vi "ADI_IMU_ADIS16448_AHRS_Madgwick.vi"(6 "Yaw Axis":enum16{"X", "Y", "Z"}(ring)=enum."Z", 8 "Reset?":bool, 9 "delta t":dbl, 10 "Beta":dbl, 11 "Data":dbl[](array[numeric])) -> (3 "Output":cluster{"Pitch":dbl, "Roll":dbl, "Yaw":dbl})   [LabVIEW 2019, in "ADIS16448_IMU.lvlib"]
uses:
  ADIS16448_IMU.lvlib
panel:
  out "Quaternion":dbl[](array[numeric])
  out "Pitch":dbl
  out "Roll":dbl
  out "Yaw":dbl
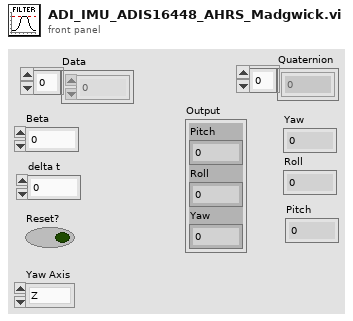
[diagram p1: front panel]
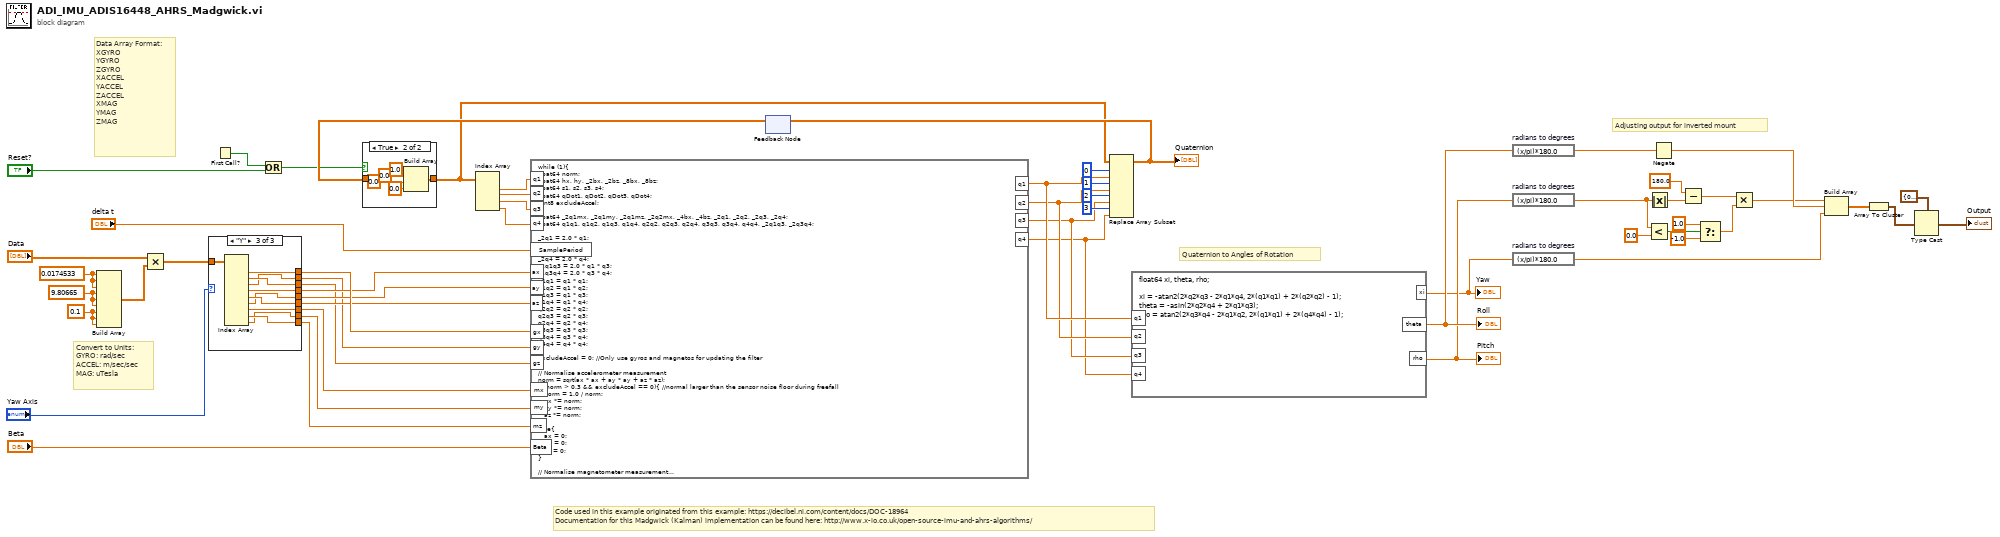
[diagram p0: block diagram]
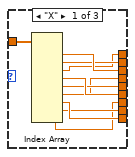
[diagram p2: hidden frame]
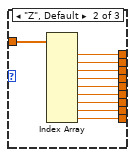
[diagram p3: hidden frame]
diagram:
  w50 = 0.1
  w51 = 9.80665
  w52 = 0.0174533
  # "Code used in this example originated from this example: https://decibel.ni.com/content/docs/DOC-18964\nDocumentation for this Madgwick (Kalman) implementation can be found here: http://www.x-io.co.uk/open-source-imu-and-ahrs-algorithms/"
  # "Quaternion to Angles of Rotation"
  # "Convert to Units:\nGYRO: rad/sec\nACCEL: m/sec/sec\nMAG: uTesla"
  # "Data Array Format:\nXGYRO\nYGYRO\nZGYRO\nXACCEL\nYACCEL\nZACCEL\nXMAG\nYMAG\nZMAG"
  # "Adjusting output for inverted mount"
  n1 = Build Array(w52, w52, w52, w51, w51, w51, w50, w50, w50) -> (w53:dbl[])
  n2 = Multiply(x="Data", y=w53) -> (x*y=w49:dbl[])
  n3 = case shown="\"Y\"" "Yaw Axis" {
    tunnel: [w63 w76 w85] -> w56
    tunnel: [w60 w75 w82] -> w55
    tunnel: w49 -> [w66 w74 w86]
    tunnel: [w57 w73 w79] -> w26
    tunnel: [w61 w72 w80] -> w25
    tunnel: [w62 w71 w81] -> w24
    tunnel: [w64 w70 w83] -> w23
    tunnel: [w65 w69 w84] -> w22
    tunnel: [w58 w68 w77] -> w21
    tunnel: [w59 w67 w78] -> w20
    frame "X" {
      n4 = Index Array(array=w66) -> (element #1=w65:dbl, element #2=w64:dbl, element #3=w63:dbl, element #4=w62:dbl, element #5=w61:dbl, element #6=w60:dbl, element #7=w59:dbl, element #8=w58:dbl, element #9=w57:dbl)  [unwired: 9 in]
    }
    frame "Z", Default {
      n5 = Index Array(array=w74) -> (element #1=w76:dbl, element #2=w70:dbl, element #3=w69:dbl, element #4=w75:dbl, element #5=w72:dbl, element #6=w71:dbl, element #7=w73:dbl, element #8=w68:dbl, element #9=w67:dbl)  [unwired: 9 in]
    }
    frame "Y" {
      n6 = Index Array(array=w86) -> (element #1=w85:dbl, element #2=w84:dbl, element #3=w83:dbl, element #4=w82:dbl, element #5=w81:dbl, element #6=w80:dbl, element #7=w79:dbl, element #8=w78:dbl, element #9=w77:dbl)  [unwired: 9 in]
    }
  }
  n7 = First Call?() -> (First Call?: T/F=w32:bool)
  n8 = Or(x=w32, y="Reset?") -> (x .or. y?=w33:bool)
  n9 = feedback #1() -> (w35:dbl[])  [unwired: 1 in]
  n10 = case shown="True" w33 {
    tunnel: w35 -> [w87 _]
    tunnel: [w87 w88] -> w34
    frame False {
    }
    frame True {
      n11 = Build Array(1.0 ("element"), 0.0 ("element"), 0.0 ("element"), 0.0 ("element")) -> (w88:dbl[])
    }
  }
  n12 = Index Array(array=w34) -> (element #1=w48:dbl, element #2=w47:dbl, element #3=w46:dbl, element #4=w45:dbl)  [unwired: 4 in]
  n13 = formula code="while (1){\nfloat64 norm;\nfloat64 hx, hy, _2bx, _2bz, _8bx, _8bz;\nfloat64 s1, s2, s3, s4;\nfloat64 qDot1, qDot2, qDot3, qDot4;\nuInt8 excludeAccel;\n\nfloat64 _2q1mx, _2q1my, _2q1mz, _2q2mx, _4bx, _4bz, _2q1, _2q2, _2q3, _2q4;\nfloat64 q1q1, q1q2, q1q3, q1q4, q2q2, q2q3, q2q4, q3q3, q3q4, q4q4, _2q1q3, _2q3q4;\n\n_2q1 = 2.0 * q1;\n_2q2 = 2.0 * q2;\n_2q3 = 2.0 * q3;\n_2q4 = 2.0 * q4;\n_2q1q3 = 2.0 * q1 * q3;\n_2q3q4 = 2.0 * q3 * q4;\nq1q1 = q1 * q1;\nq1q2 = q1 * q2;\nq1q3 = q1 * q3;\nq1q4 = q1 * q4;\nq2q2 = q2 * q2;\nq2q3 = q2 * q3;\nq2q4 = q2 * q4;\nq3q3 = q3 * q3;\nq3q4 = q3 * q4;\nq4q4 = q4 * q4;\n\nexcludeAccel = 0; //Only use gyros and magnetos for updating the filter\n\n// Normalise accelerometer measurement\nnorm = sqrt(ax * ax + ay * ay + az * az);\nif (norm > 0.3 && excludeAccel == 0){ //normal larger than the sensor noise floor during freefall\n   norm = 1.0 / norm; \n   ax *= norm;\n   ay *= norm;\n   az *= norm;\n}\nelse{\n   ax = 0;\n   ay = 0;\n   az = 0;\n}\n\n// Normalise magnetometer measurement\nnorm = sqrt(mx * mx + my * my + mz * mz);\nif (norm > 0.0){\n   norm = 1.0 / norm;\n   mx *= norm;\n   my *= norm;\n   mz *= norm;\n}\nelse{\n  break; //something is wrong with the magneto readouts\n}\n\n// Reference direction of Earth's magnetic field\n_2q1mx = 2 * q1 * mx;\n_2q1my = 2 * q1 * my;\n_2q1mz = 2 * q1 * mz;\n_2q2mx = 2 * q2 * mx;\n\nhx = mx * q1q1 - _2q1my * q4 + _2q1mz * q3 + mx * q2q2 + _2q2 * my * q3 + _2q2 * mz * q4 - mx * q3q3 - mx * q4q4;\nhy = _2q1mx * q4 + my * q1q1 - _2q1mz * q2 + _2q2mx * q3 - my * q2q2 + my * q3q3 + _2q3 * mz * q4 - my * q4q4;\n_2bx = sqrt(hx * hx + hy * hy);\n_2bz = -_2q1mx * q3 + _2q1my * q2 + mz * q1q1 + _2q2mx * q4 - mz * q2q2 + _2q3 * my * q4 - mz * q3q3 + mz * q4q4;\n_4bx = 2.0 * _2bx;\n_4bz = 2.0 * _2bz;\n_8bx = 2.0 * _4bx;\n_8bz = 2.0 * _4bz;\n\n// Gradient descent algorithm corrective step\ns1 = -_2q3 * (2.0 * q2q4 - _2q1q3 - ax) + _2q2 * (2.0 * q1q2 + _2q3q4 - ay) - _4bz * q3 * (_4bx * (0.5 - q3q3 - q4q4) + _4bz * (q2q4 - q1q3) - mx) + (-_4bx * q4 + _4bz * q2) * (_4bx * (q2q3 - q1q4) + _4bz * (q1q2 + q3q4) - my) + _4bx * q3 * (_4bx * (q1q3 + q2q4) + _4bz * (0.5 - q2q2 - q3q3) - mz);\ns2 = _2q4 * (2.0 * q2q4 - _2q1q3 - ax) + _2q1 * (2.0 * q1q2 + _2q3q4 - ay) - 4.0 * q2 * (1.0 - 2.0 * q2q2 - 2.0 * q3q3 - az) + _4bz * q4 * (_4bx * (0.5 - q3q3 - q4q4) + _4bz * (q2q4 - q1q3) - mx) + (_4bx * q3 + _4bz * q1) * (_4bx * (q2q3 - q1q4) + _4bz * (q1q2 + q3q4) - my) + (_4bx * q4 - _8bz * q2) * (_4bx * (q1q3 + q2q4) + _4bz * (0.5 - q2q2 - q3q3) - mz);\ns3 = -_2q1 * (2.0 * q2q4 - _2q1q3 - ax) + _2q4 * (2.0 * q1q2 + _2q3q4 - ay) - 4.0 * q3 * (1.0 - 2.0 * q2q2 - 2.0 * q3q3 - az) + (-_8bx * q3 - _4bz * q1) * (_4bx * (0.5 - q3q3 - q4q4) + _4bz * (q2q4 - q1q3) - mx) + (_4bx * q2 + _4bz * q4) * (_4bx * (q2q3 - q1q4) + _4bz * (q1q2 + q3q4) - my) + (_4bx * q1 - _8bz * q3) * (_4bx * (q1q3 + q2q4) + _4bz * (0.5 - q2q2 - q3q3) - mz);\ns4 = _2q2 * (2.0 * q2q4 - _2q1q3 - ax) + _2q3 * (2.0 * q1q2 + _2q3q4 - ay) + (-_8bx * q4 + _4bz * q2) * (_4bx * (0.5 - q3q3 - q4q4) + _4bz * (q2q4 - q1q3) - mx) + (-_4bx * q1 + _4bz * q3) * (_4bx * (q2q3 - q1q4) + _4bz * (q1q2 + q3q4) - my) + _4bx * q2 * (_4bx * (q1q3 + q2q4) + _4bz * (0.5 - q2q2 - q3q3) - mz);\n\nnorm = sqrt(s1 * s1 + s2 * s2 + s3 * s3 + s4 * s4);\nif (norm > 0.0){\n   norm = 1.0 / norm;  //normalise gradient step\n   s1 *= norm;\n   s2 *= norm;\n   s3 *= norm;\n   s4 *= norm;\n}\nelse{\n   break;\n}\n\n// Compute rate of change of quaternion\nqDot1 = 0.5 * (-q2 * gx - q3 * gy - q4 * gz) - Beta * s1;\nqDot2 = 0.5 * (q1 * gx + q3 * gz - q4 * gy) - Beta * s2;\nqDot3 = 0.5 * (q1 * gy - q2 * gz + q4 * gx) - Beta * s3;\nqDot4 = 0.5 * (q1 * gz + q2 * gy - q3 * gx) - Beta * s4;\n\n// Integrate to yield quaternion\nq1 += qDot1 * SamplePeriod;\nq2 += qDot2 * SamplePeriod;\nq3 += qDot3 * SamplePeriod;\nq4 += qDot4 * SamplePeriod;\n\nnorm = sqrt(q1 * q1 + q2 * q2 + q3 * q3 + q4 * q4);\nif (norm > 0.0){\n   norm = 1.0 / norm;  //normalise quaternion\n   q1 = q1 * norm;\n   q2 = q2 * norm;\n   q3 = q3 * norm;\n   q4 = q4 * norm;\n}\nbreak;\n}"("q1"=w48, "gx"=w56, "gy"=w23, "gz"=w22, "ax"=w55, "ay"=w25, "az"=w24, "mx"=w26, "my"=w21, "mz"=w20, "SamplePeriod"="delta t", "Beta"="Beta", "q2"=w47, "q3"=w46, "q4"=w45) -> ("q1"=w39:dbl, "q2"=w38:dbl, "q3"=w37:dbl, "q4"=w36:dbl)
  n14 = Replace Array Subset(array=w34, new element #1=w39, index #1=0 ("index"), new element #2=w38, index #2=1 ("index"), new element #3=w37, index #3=2 ("index"), new element #4=w36, index #4=3 ("index")) -> (w40:dbl[])
  "Quaternion" <- w40
  n15 = feedback-in #1(w40) -> ()
  n16 = formula code="float64 xi, theta, rho;\n\nxi = -atan2(2*q2*q3 - 2*q1*q4, 2*(q1*q1) + 2*(q2*q2) - 1);\ntheta = -asin(2*q2*q4 + 2*q1*q3);\nrho = atan2(2*q3*q4 - 2*q1*q2, 2*(q1*q1) + 2*(q4*q4) - 1);"("q1"=w39, "q2"=w38, "q3"=w37, "q4"=w36) -> ("xi"=w28:dbl, "theta"=w30:dbl, "rho"=w29:dbl)
  "Yaw" <- w28
  "Roll" <- w30
  "Pitch" <- w29
  n17 = expression code="(x/pi)*180.0" "radians to degrees"(w30) -> (w10:dbl)
  n18 = expression code="(x/pi)*180.0" "radians to degrees"(w29) -> (w17:dbl)
  n19 = expression code="(x/pi)*180.0" "radians to degrees"(w28) -> (w27:dbl)
  n20 = Less?(x=w17, y=0.0) -> (x < y?=w15:bool)
  n21 = Absolute Value(x=w17) -> (abs(x)=w19:dbl)
  n22 = Negate(x=w10) -> (-x=w9:dbl)
  n23 = Subtract(x=180.0 ("y"), y=w19) -> (x-y=w12:dbl)
  n24 = Select(t=1.0, s=w15, f=-1.0) -> (s? t:f=w11:dbl)
  n25 = Multiply(x=w12, y=w11) -> (x*y=w8:dbl)
  n26 = Build Array(w8, w9, w27) -> (w3:dbl[])
  n27 = Array To Cluster(array=w3) -> (cluster=w4:cluster{"[0]":dbl, "[1]":dbl, "[2]":dbl})
  n28 = Type Cast(type=cluster{"Pitch":dbl, "Roll":dbl, "Yaw":dbl} {"Pitch"=0.0, "Roll"=0.0, "Yaw"=0.0} ("IMU AHRS"), x=w4) -> (*(type *) &x=→"Output":cluster{"Pitch":dbl, "Roll":dbl, "Yaw":dbl})
